vi "cancel subscription.vi"(9 "queue":refnum<class "identifying queue.lvclass">, 10 "pattern":string, 11 "registered subscriptions in":T1) -> (3 "registered subscriptions out":T1)   [LabVIEW 2015, in "publisher.lvclass"]
uses:
  publisher.lvclass
  registered subscriptions.ctl
  communicator queue/identifying queue.lvclass
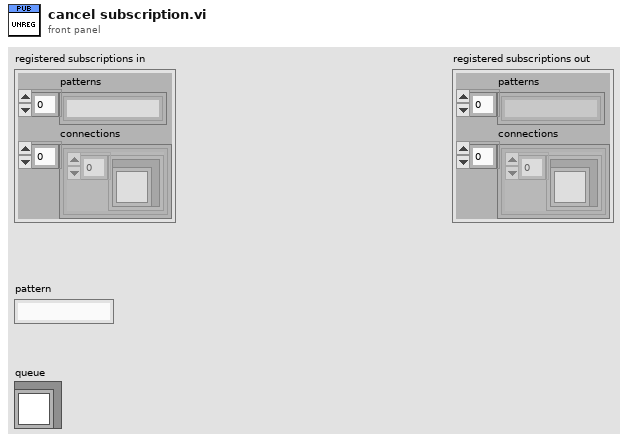
[diagram p1: front panel]
types:
  T1 = typedef "publisher.lvclass/registered subscriptions.ctl" = cluster{"patterns":string[], "connections":cluster{"connections":refnum<class "identifying queue.lvclass">[]}[]}
  T2 = cluster{"connections":refnum<class "identifying queue.lvclass">[]}[]
  T3 = cluster{"connections":refnum<class "identifying queue.lvclass">[]}
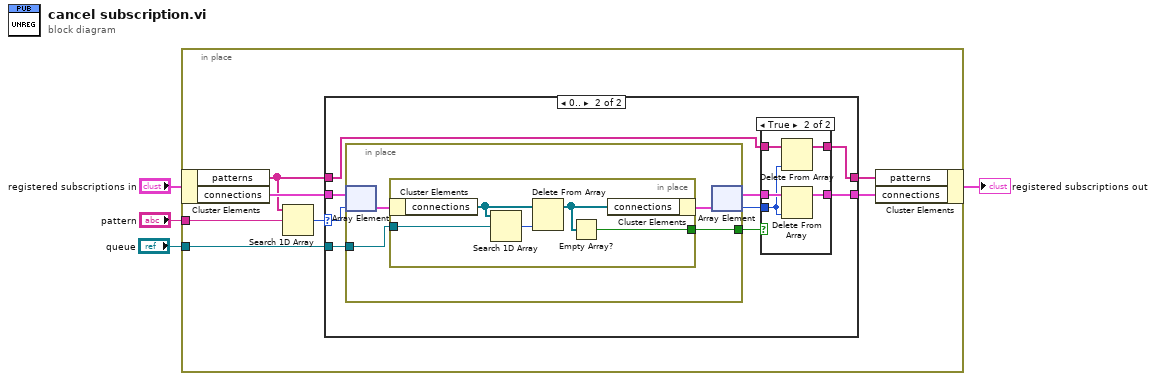
[diagram p0: block diagram]
diagram:
  n1 = in-place {
    in-place-border: "pattern" -> [w5]
    in-place-border: "queue" -> [w6]
    n2 = in-place-cluster #1("registered subscriptions in") -> ("patterns"=w8:string[], "connections"=w10:T2)
    n3 = Search 1D Array(1D array=w8, element=w5) -> (index of element=w11:i32)  [unwired: 1 in]
    n4 = case shown="0.." w11 {
      selector: w11 -> [_ w21]
      tunnel: w10 -> [w12 w22]
      tunnel: [w12 w15] -> w9
      tunnel: w8 -> [w13 w18]
      tunnel: [w13 w17] -> w7
      tunnel: w6 -> [_ w20]
      frame ..-1 {
      }
      frame 0.. {
        n5 = in-place {
          in-place-border: w20 -> [w31]
          in-place-border: [w30] -> w19
          n6 = in-place-array #2(w22, w21) -> (w33:T3)
          n7 = in-place {
            in-place-border: w31 -> [w38]
            in-place-border: [w34] -> w30
            n8 = in-place-cluster #3(w33) -> ("connections"=w37:refnum<class "identifying queue.lvclass">[])
            n9 = Search 1D Array(1D array=w37, element=w38) -> (index of element=w36:i32)  [unwired: 1 in]
            n10 = Delete From Array(array=w37, index=w36) -> (array with subset deleted=w35:refnum<class "identifying queue.lvclass">[])  [unwired: 1 in, 1 out]
            n11 = Empty Array?(array=w35) -> (empty?=w34:bool)
            n12 = in-place-cluster #3("connections"=w35) -> (w32:T3)
          }
          n13 = in-place-array #2(w32) -> (w16:T2, w14:i32)
        }
        n14 = case shown="True" w19 {
          tunnel: [w24 w27] -> w17
          tunnel: w18 -> [w24 w28]
          tunnel: w16 -> [w23 w29]
          tunnel: [w23 w26] -> w15
          tunnel: w14 -> [_ w25]
          frame False {
          }
          frame True {
            n15 = Delete From Array(array=w28, index=w25) -> (array with subset deleted=w27:string[])  [unwired: 1 in, 1 out]
            n16 = Delete From Array(array=w29, index=w25) -> (array with subset deleted=w26:T2)  [unwired: 1 in, 1 out]
          }
        }
      }
    }
    n17 = in-place-cluster #1("patterns"=w7, "connections"=w9) -> (→"registered subscriptions out":T1)
  }
